vi "Write Data.vi"(8 "error in (no error)":errorcluster, 10 "PAS Data":refnum<class "PAS Data.lvclass">, 11 "PAS in":refnum<class "PAS.lvclass">) -> (0 "error out":errorcluster, 3 "PAS out":refnum<class "PAS.lvclass">)   [LabVIEW 2014, in "PAS.lvclass"]
uses:
  PAS.lvclass
  Data/Main/PAS Data.lvclass
  PAS.lvclass/PAS.ctl
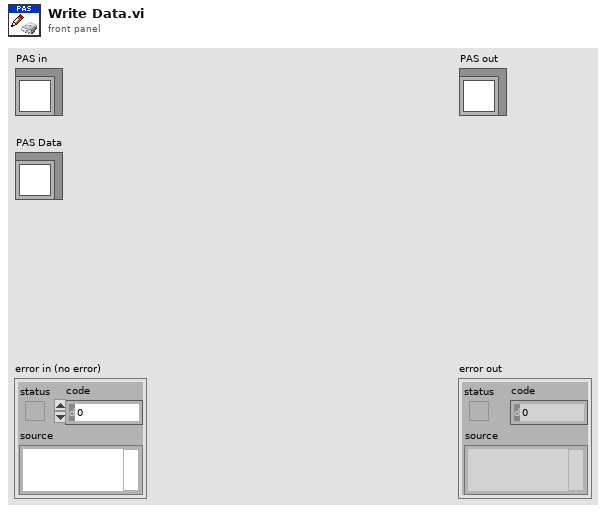
[diagram p1: front panel]
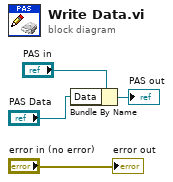
[diagram p0: block diagram]
diagram:
  n1 = Bundle By Name(cluster="PAS in", "Data"="PAS Data") -> (→"PAS out":refnum<class "PAS.lvclass">)
  "error out" <- "error in (no error)"
